vi "Przesuwnik_fazowy.vi"(11 "Parametry_cosinusow":T1) -> (3 "Parametry_cosinusow\nprzesuniete_w_fazie":T2[](array[typedef]))   [LabVIEW 2020]
doc: "VI przesuwa w fazie o -90 stopni (-pi/2 w radianach) sygnaly sinusoidalne, z ktorych sklada sie sygnal modulujacy."
uses:
  Kontrolki/Parametry_cosinusa.ctl
  Kontrolki/Parametry_cosinusow.ctl
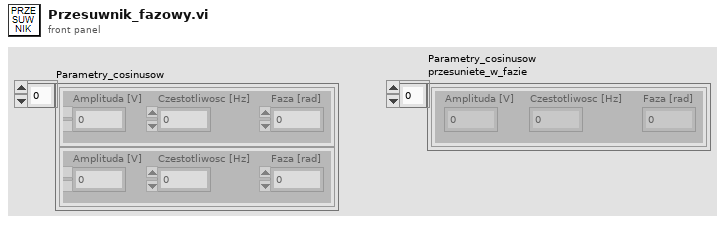
[diagram p1: front panel]
types:
  T1 = typedef "Parametry_cosinusow.ctl" = T2[]
  T2 = typedef "Parametry_cosinusa.ctl" = cluster{"Amplituda [V]":dbl, "Czestotliwosc [Hz] ":dbl, "Faza [rad]":dbl}
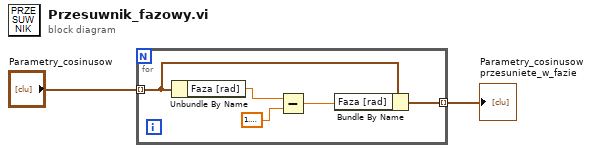
[diagram p0: block diagram]
diagram:
  n1 = for {
    tunnel: "Parametry_cosinusow" -> [w5] mode=indexing
    tunnel: [w3] -> w2 mode=indexing
    n2 = Unbundle By Name(w5) -> ("Faza [rad]"=w6:dbl)
    n3 = Subtract(x=w6, y=1.5707963267948966) -> (x-y=w4:dbl)
    n4 = Bundle By Name(cluster=w5, "Faza [rad]"=w4) -> (w3:T2)
  }
  "Parametry_cosinusow\nprzesuniete_w_fazie" <- w2
